vi "Get SICK (Only) Data.vi"(8 "error in":errorcluster, 11 "SICK Only ref in":T2) -> (0 "error out":errorcluster, 2 "SICK Data":T1, 3 "SICK Only ref out":T2)   [LabVIEW 2009]
uses:
  <vilib>/rvi/interface/nirviMethod/nirviMethod.xnode
  SICK Only FPGA Ref.ctl
  FPGA Bitfiles/Q_IGVC_2010.lvproj_FPGA Target_SICK Only.vi.lvbitx
  TypeDefs/Sensor Typedefs/SICK Array.ctl
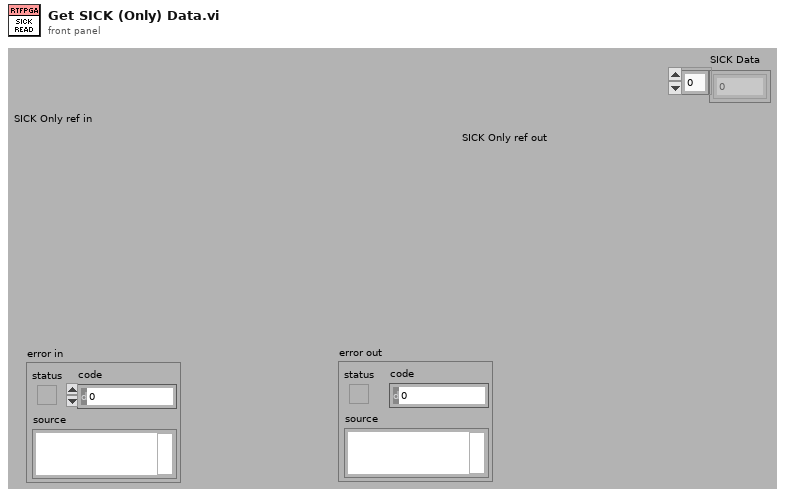
[diagram p1: front panel]
types:
  T1 = typedef "SICK Array.ctl" = u16[]
  T2 = typedef "SICK Only FPGA Ref.ctl" = refnum<k20>
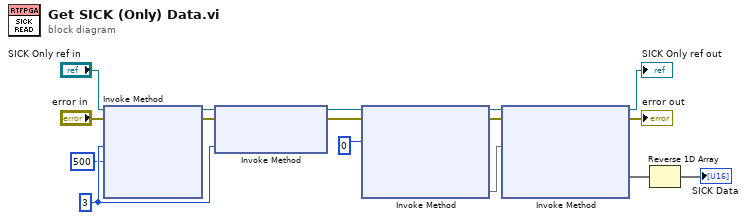
[diagram p0: block diagram]
diagram:
  w8 = 3 ("IRQ Number(s)")
  n1 = xnode "Invoke Method"("FPGA VI Reference In"="SICK Only ref in", "error in"="error in", "IRQ Number(s)"=w8, "Timeout (ms)"=500) -> ("FPGA VI Reference Out"=w10:T2, "error out"=w9:errorcluster)  [unwired: 2 out]
  n2 = xnode "Invoke Method"("FPGA VI Reference In"=w10, "error in"=w9, "IRQ Number(s)"=w8) -> ("FPGA VI Reference Out"=w3:T2, "error out"=w2:errorcluster)
  n3 = xnode "Invoke Method"("FPGA VI Reference In"=w3, "error in"=w2, "Number of Elements"=u32 0) -> ("FPGA VI Reference Out"=w4:T2, "error out"=w5:errorcluster, "Elements Remaining"=w7)  [unwired: 1 in, 1 out]
  n4 = xnode "Invoke Method"("FPGA VI Reference In"=w4, "error in"=w5, "Number of Elements"=w7) -> ("FPGA VI Reference Out"=→"SICK Only ref out":T2, "error out"=→"error out":errorcluster, "Data"=w14:void[])  [unwired: 1 in, 1 out]
  n5 = Reverse 1D Array(array=w14) -> (reversed array=→"SICK Data":void[])
